vi "SA Math - ReSample ONE Signal.vi"(0 "wForm IN":waveform(dbl), 5 "error in (no error)":errorcluster, 7 "New Fs":dbl, 8 "Anotate Signal Name":bool=TRUE) -> (13 "Signal Resampled?":bool, 14 "wForm OUT":waveform(dbl), 19 "error out":errorcluster)   [LabVIEW 2022 SP3, in "GSwFormDSP.lvclass"]
uses:
  GSwFormDSP.lvclass
  functions/Attribute List.ctl
  functions/Attribute Options.ctl
  <vilib>/Analysis/2dsp.llb/Resample (constant to constant,single -channel).vi
  <vilib>/Analysis/NI_AALPro.lvlib
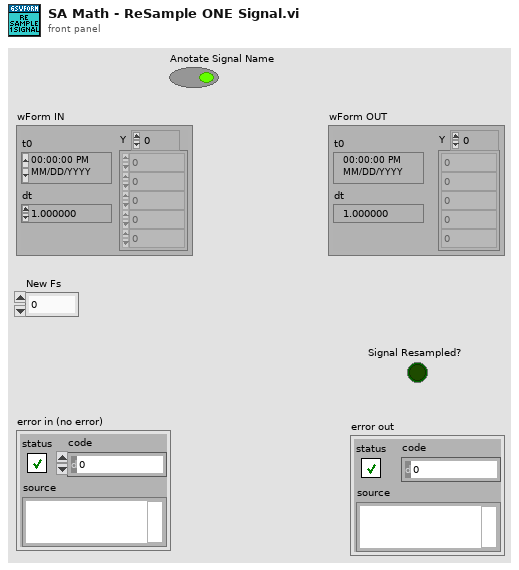
[diagram p1: front panel]
types:
  T1 = cluster{"alias rejection (dB)":dbl, "normalized bandwidth":dbl}
  T2 = typedef "GSwFormDSP.lvclass/Attribute Options.ctl" = enum16{"Append to Attribute using \"( )\"", "Replace Attribute Value"}
  T3 = typedef "GSwFormDSP.lvclass/Attribute List.ctl" = string
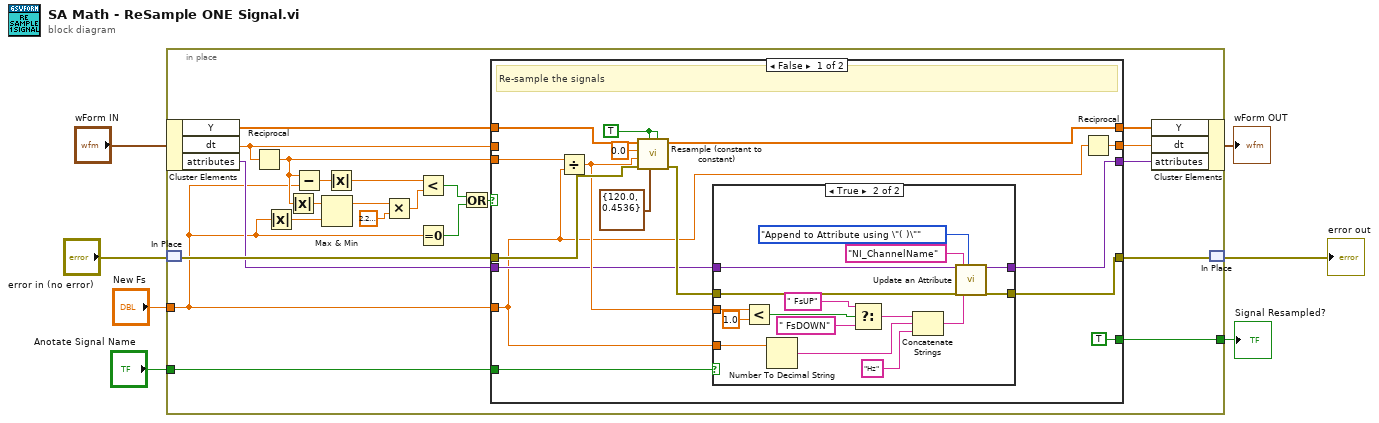
[diagram p0: block diagram]
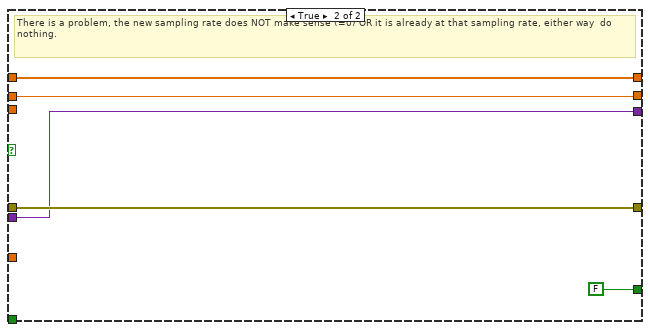
[diagram p3: hidden frame]
diagram:
  n1 = in-place {
    in-place-border: "New Fs" -> [w15]
    in-place-border: "Anotate Signal Name" -> [w20]
    in-place-border: [w18] -> w1
    n2 = in-place-cluster #1("wForm IN") -> ("Y"=w29:dbl[], "dt"=w25:dbl, "attributes"=w19:variant)
    n3 = in-place-match #2("error in (no error)") -> (w22:errorcluster)
    n4 = Reciprocal(x=w25) -> (1/x=w16:dbl)
    n5 = Absolute Value(x=w15) -> (abs(x)=w13:dbl)
    n6 = Absolute Value(x=w16) -> (abs(x)=w14:dbl)
    n7 = Subtract(x=w16, y=w15) -> (x-y=w17:dbl)
    n8 = Max & Min(x=w14, y=w13) -> (max(x,y)=w11:dbl)  [unwired: 1 out]
    n9 = Absolute Value(x=w17) -> (abs(x)=w10:dbl)
    n10 = Multiply(x=w11, y=2.220446049250313e-16) -> (x*y=w9:dbl)
    n11 = Less?(x=w10, y=w9) -> (x < y?=w8:bool)
    n12 = Equal To 0?(x=w15) -> (x = 0?=w24:bool)
    n13 = Or(x=w8, y=w24) -> (x .or. y?=w23:bool)
    n14 = case shown="False" w23 {
      tunnel: w29 -> [w42 w68]
      tunnel: w25 -> [_ w67]
      tunnel: [w41 w67] -> w28
      tunnel: [w39 w68] -> w27
      tunnel: [w32 w65] -> w26
      tunnel: w15 -> [w30 _]
      tunnel: w16 -> [w38 _]
      tunnel: w22 -> [w40 w66]
      tunnel: [w34 w66] -> w21
      tunnel: w20 -> [w36 _]
      tunnel: w19 -> [w33 w65]
      tunnel: [TRUE ("Signal Resampled?") FALSE ("Signal Resampled?")] -> w18
      frame False {
        w45 = TRUE
        # "Re-sample the signals"
        n15 = Divide(x=w38, y=w30) -> (x/y=w37:dbl)
        n16 = call-poly <vilib>:"Resample (constant to constant).vi"("anti-aliasing?"=w45, "FIR filter specifications"=T1 {"alias rejection (dB)"=120.0, "normalized bandwidth"=0.4536}, "reset?"=w45, "error in (no error)"=w40, "dt"=w37, "delay"=0.0, "X"=w42) -> ("error out"=w35:errorcluster, "Y"=w39:dbl[])  [unwired: 2 in, 1 out]
        n17 = case shown="True" w36 {
          tunnel: w30 -> [_ w48]
          tunnel: w37 -> [_ w60]
          tunnel: w35 -> [w47 w54]
          tunnel: [w47 w53] -> w34
          tunnel: w33 -> [w46 w52]
          tunnel: [w46 w51] -> w32
          frame False {
          }
          frame True {
            n18 = Less?(x=w60, y=1.0) -> (x < y?=w59:bool)
            n19 = Number To Decimal String(number=w48) -> (decimal integer string=w63:string)  [unwired: 1 in]
            n20 = Select(t=" FsUP" ("string"), s=w59, f=" FsDOWN" ("string")) -> (s? t:f=w56:string)
            n21 = Concatenate Strings(w56, w63, "Hz" ("string")) -> (w55:string)
            n22 = call "Update an Attribute.vi"("attributes in"=w52, "error in (no error)"=w54, "Attribute List"=T3 "NI_ChannelName", "Attribute Value"=w55, "Attribute Option"=Attribute_Options."Append to Attribute using \"( )\"") -> ("attributes out"=w51:variant, "error out"=w53:errorcluster)  [unwired: 13 in]
          }
        }
        n23 = Reciprocal(x=w30) -> (1/x=w41:dbl)
      }
      frame True {
        # "There is a problem, the new sampling rate does NOT make sense (=0) OR it is already at that sampling rate, either way  do nothing."
      }
    }
    n24 = in-place-cluster #1("Y"=w27, "dt"=w28, "attributes"=w26) -> (→"wForm OUT":waveform(dbl))
    n25 = in-place-match #2(w21) -> (→"error out":errorcluster)
  }
  "Signal Resampled?" <- w1
